vi "ExitSubroutine.vi"(8 "error in (no error)":errorcluster, 11 "AutoSubroutine in":refnum<class "AutoSubroutine.lvclass">) -> (0 "error out":errorcluster, 3 "AutoSubroutine out":refnum<class "AutoSubroutine.lvclass">)   [LabVIEW 2017, in "AutoSubroutine.lvclass"]
uses:
  AutoSubroutine.lvclass
  AutoSubroutine.lvclass/AutoSubroutine.ctl
  Subsystem/Subsystem.lvclass
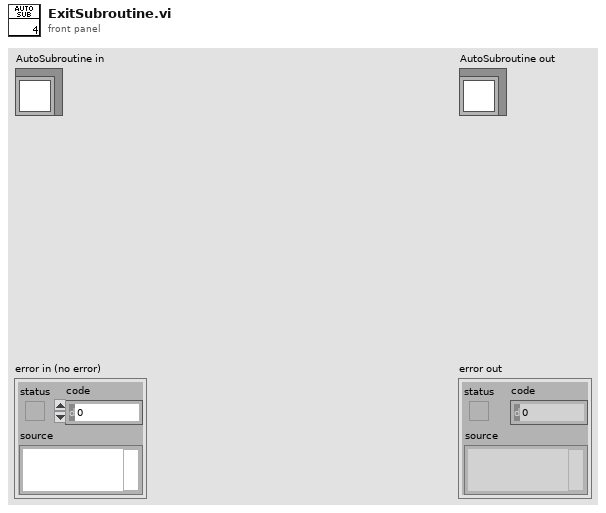
[diagram p1: front panel]
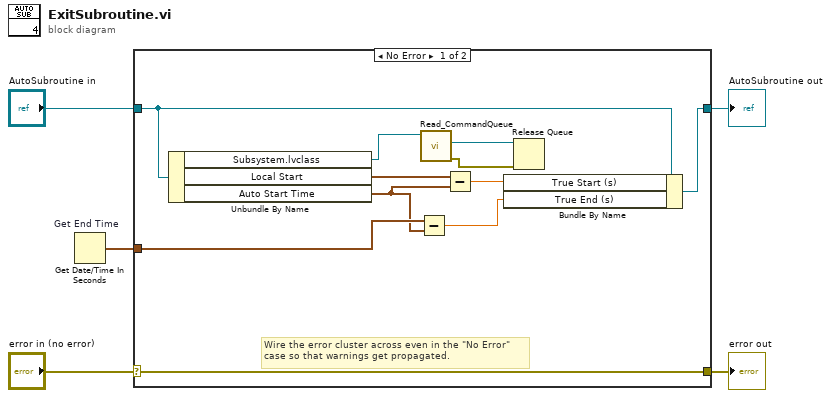
[diagram p0: block diagram]
diagram:
  n1 = Get Date/Time In Seconds "Get End Time"() -> (seconds since 1Jan1904=w1:timestamp)
  n2 = case shown="No Error" "error in (no error)" {
    selector: "error in (no error)" -> [w16 w18]
    tunnel: [w16 w18] -> w4
    tunnel: [w14 w17] -> w2
    tunnel: "AutoSubroutine in" -> [w15 w17]
    tunnel: w1 -> [w11 _]
    frame No Error {
      # "Wire the error cluster across even in the \"No Error\"\ncase so that warnings get propagated."
      n3 = Unbundle By Name(w15) -> ("Subsystem.lvclass"=w8:refnum<class "Subsystem.lvclass">, "Local Start"=w13:timestamp, "Auto Start Time"=w10:timestamp)
      n4 = Subtract(x=w11, y=w10) -> (x-y=w9:dbl)
      n5 = call-dynamic "Read_CommandQueue.vi"("Subsystem in"=w8) -> ("error out"=w6:errorcluster, "Command Queue"=w7:refnum<queue>)  [unwired: 8 in, 1 out]
      n6 = Subtract(x=w13, y=w10) -> (x-y=w12:dbl)
      n7 = Bundle By Name(cluster=w15, "True Start (s)"=w12, "True End (s)"=w9) -> (w14:refnum<class "AutoSubroutine.lvclass">)
      n8 = Release Queue(queue=w7, error in (no error)=w6) -> ()  [unwired: 1 in, 3 out]
    }
    frame Error {
    }
  }
  "error out" <- w4
  "AutoSubroutine out" <- w2
